vi "Ackermann_FullStochastic_StateSpace.vi"() -> ()   [LabVIEW 2017]
uses:
  <vilib>/Simulation/Scripting/Companion Diagram/SimConfigNode/SimParams.ctl
  <vilib>/Simulation/Scripting/Companion Diagram/SimConfigNode/_simSolvers.ctl
  <vilib>/Simulation/Implementation/Shared/SIMSCR Execution Mode.ctl
  <vilib>/Simulation/Param Hierarchy/Typedefs/SIMPH Param Control Actions.ctl
  <vilib>/Simulation/Implementation/Shared/NILVSim_ParamChanged.vi
  <vilib>/Simulation/Implementation/Shared/NILVSIM_BeginStep.vi
  <vilib>/Simulation/SignalDisplay/Implementation/NILVSim Time Waveform.llb/SIM Time Waveform (vector).vi
  <vilib>/Simulation/Implementation/Shared/NILVSim_Manager.vi
  <vilib>/Utility/error.llb/Clear Errors.vi
  <vilib>/Simulation/Implementation/Shared/NILVSim_FinalizeModel.vi
  <vilib>/Simulation/Implementation/Shared/SIM Unbundle Sim Info.vi
  <vilib>/Simulation/Implementation/Shared/NILVSim_Initialize.vi
  <vilib>/Simulation/Utility/Implementation/NILVSim Get Time and IsAcceptedStep.vi
  <vilib>/Simulation/DiscreteLinear/Implementation/NILVSim Discrete Stochastic State Space.llb/SIM Discrete Stochastic State Space External Indirect Distributor Sim.vi
  <vilib>/Simulation/DiscreteLinear/Implementation/NILVSim Discrete Stochastic State Space.llb/SIM Discrete Stochastic State Space External Indirect Collector Sim.vi
  <vilib>/Simulation/Implementation/Shared/SIMSH Read Queue.vi
  <vilib>/Simulation/Implementation/Shared/NILVSim_GetModelError.vi
  <vilib>/Simulation/Implementation/Shared/SIM Bundle Sim Info.vi
  <vilib>/Simulation/Scripting/Companion Diagram/SimConfigNode/SimDog.xnode
  <vilib>/Simulation/Implementation/XNodeFramework/SimXNode/SimX.xnode
  <vilib>/Simulation/DiscreteLinear/Implementation/NILVSim Discrete Stochastic State Space.llb/NILVSim Discrete Stochastic State Space External Indirect Sim.vi
  <vilib>/Simulation/Implementation/Shared/NI_SIM_Implementation.lvlib
panel:
  out "State Trajectory Graph- Y":cluster{"time":dbl[], dbl[]}[](graph)
  out "State Trajectory Graph- X":cluster{"time":dbl[], dbl[]}[](graph)
  out "State Trajectory Graph- Z":cluster{"time":dbl[], dbl[]}[](graph)
  out "State Trajectory Graph- Phi":cluster{"time":dbl[], dbl[]}[](graph)
  out "State Trajectory Graph- Psi":cluster{"time":dbl[], dbl[]}[](graph)
  out "State Trajectory Graph- Theta":cluster{"time":dbl[], dbl[]}[](graph)
  out "Gain Y":dbl[](array[numeric]) format="%.3f"
  out "Gain X":dbl[](array[numeric]) format="%.3f"
  out "Gain":dbl[](array[numeric]) format="%.3f"
  in  "Phi_rate":dbl
  in  "Theta_rate":dbl
  out "Psi-SSS":picture
  out "Closed-Loop Step Response- Psi":cluster{"time":dbl[], dbl[]}[](graph)
  in  "Imaginary 6":dbl(knob)=-10.013861291935129 scale=0.0..-20.0 scale format="%#_4g"
  in  "Real 6":dbl(knob)=-3.4076115316471642 scale=0.0..-22.0 scale format="%#_4g"
  in  "Psi-Setpoints":dbl[](array[numeric])
  out "State x(k) Psi":dbl[](array[numeric])
  out "Psi":dbl[](array[numeric])
  out "Ux-Phi 4":dbl[](array[numeric]) format="%#.2g"
  out "Waveform Psi":waveform(dbl)[](graph)
  out "theta-SSS":picture
  out "Closed-Loop Step Response- Theta":cluster{"time":dbl[], dbl[]}[](graph)
  in  "Imaginary 5":dbl(knob)=-10.013861291935129 scale=0.0..-20.0 scale format="%#_4g"
  in  "Real 5":dbl(knob)=-3.4076115316471642 scale=0.0..-22.0 scale format="%#_4g"
  out "Theta-Setpoints":dbl[](array[numeric])
  out "State x(k) Theta":dbl[](array[numeric])
  out "Theta":dbl[](array[numeric])
  out "Ux-Phi 3":dbl[](array[numeric]) format="%#.2g"
  out "Waveform Theta":waveform(dbl)[](graph)
  out "Phi-SSS":picture
  out "Closed-Loop Step Response- Phi":cluster{"time":dbl[], dbl[]}[](graph)
  in  "Imaginary 4":dbl(knob)=-10.013861291935129 scale=0.0..-20.0 scale format="%#_4g"
  in  "Real 4":dbl(knob)=-3.4076115316471642 scale=0.0..-22.0 scale format="%#_4g"
  out "Phi-Setpoints":dbl[](array[numeric])
  out "State x(k) Phi":dbl[](array[numeric])
  out "Phi":dbl[](array[numeric])
  out "Ux-Phi 2":dbl[](array[numeric]) format="%#.2g"
  out "Waveform Phi":waveform(dbl)[](graph)
  out "Y-SSS":picture
  out "Closed-Loop Step Response- Y":cluster{"time":dbl[], dbl[]}[](graph)
  in  "Imaginary 3":dbl(knob)=-10.013861291935129 scale=0.0..-20.0 scale format="%#_4g"
  in  "Real 3":dbl(knob)=-3.4076115316471642 scale=0.0..-22.0 scale format="%#_4g"
  in  "Y-Setpoints":dbl[](array[numeric])
  out "State x(k) Y":dbl[](array[numeric])
  out "Y":dbl[](array[numeric])
  out "Uy-Theta":dbl[](array[numeric]) format="%#.2g"
  out "Waveform Y":waveform(dbl)[](graph)
  out "X-SSS":picture
  out "Closed-Loop Step Response- X":cluster{"time":dbl[], dbl[]}[](graph)
  in  "Imaginary 2":dbl(knob)=-10.013861291935129 scale=0.0..-20.0 scale format="%#_4g"
  in  "Real 2":dbl(knob)=-3.4076115316471642 scale=0.0..-22.0 scale format="%#_4g"
  in  "X-Setpoints":dbl[](array[numeric])
  out "State x(k) X":dbl[](array[numeric])
  out "X":dbl[](array[numeric])
  out "Ux-Phi":dbl[](array[numeric]) format="%#.2g"
  out "Waveform X":waveform(dbl)[](graph)
  out "Equation":picture
  in  "reset?":bool
  out "Closed-Loop Step Response":cluster{"time":dbl[], dbl[]}[](graph)
  in  "Imaginary":dbl(knob)=-10.013861291935129 scale=0.0..-20.0 scale format="%#_4g"
  in  "Real":dbl(knob)=-3.4076115316471642 scale=0.0..-22.0 scale format="%#_4g"
  in  "Alt-Setpoints":dbl[](array[numeric])
  out "State x(k) Alt":dbl[](array[numeric])
  out "Altitude":dbl[](array[numeric])
  out "ut":dbl[](array[numeric]) format="%#.2g"
  out "Waveform Altitude":waveform(dbl)[](graph)
  # "I"
  # "R"
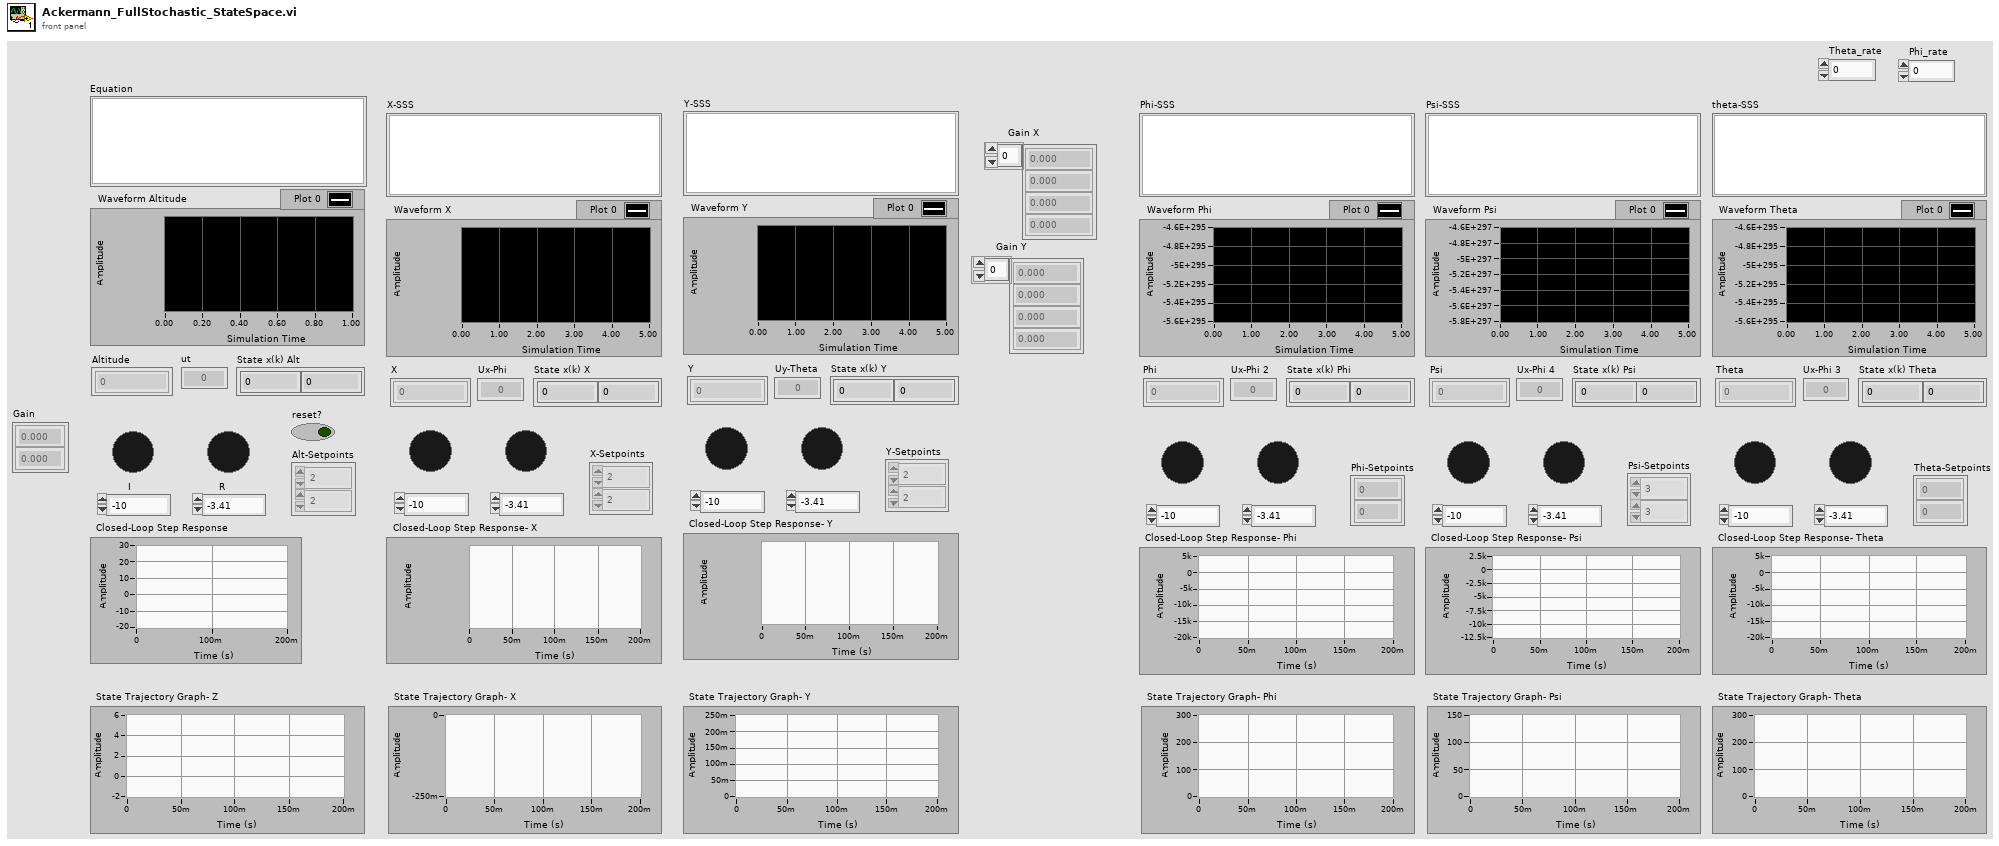
[diagram p1: front panel]
types:
  T1 = typedef "NI_LinSys_Model Typedefs.lvlib/CD State Space Model (MIMO).ctl" = cluster{"properties":T2, "A":dbl[][], "B":dbl[][], "C":dbl[][], "D":dbl[][], "StateNames":string[], "Transport Delay":dbl[][]}
  T2 = typedef "NI_LinSys_Model Typedefs.lvlib/CD General Elements.ctl" = cluster{"Model name":string, "Input names":string[], "Output names":string[], "Input Delays":dbl[], "Output Delays":dbl[], "Sampling Time":dbl, "Notes":string}
  T3 = typedef "NI_CD_Stochastic Systems.lvlib/cd_Stochastic State-Space Model.ctl" = cluster{"Sampling Time (s)":dbl, "G":dbl[][], "B":dbl[][], "A":dbl[][], "C":dbl[][], "D":dbl[][], "H":dbl[][]}
  T4 = typedef "SIMSCR Execution Mode.ctl" = enum16{"Simulate to Completion", "Single Time-Step Simulation (Fixed Step Only)"}
  T5 = typedef "SIMPH Param Control Actions.ctl" = enum16{"get params", "set params"}
  T6 = typedef "SimParams.ctl" = cluster{"Initial Time (s)":dbl, "Final Time (s)":dbl, "Step Size (s)":dbl, "ODE Solver":T7, "Minimum Step Size (s)":dbl, "Maximum Step Size (s)":dbl, "Relative Tolerance":dbl, "Absolute Tolerance":dbl, "Software Timing":bool, "Initial Step Size (s)":dbl, "Automatic Fixed Step Size?":bool, "Automatic Discrete Step Size?":bool, "Discrete Step Size (s)":dbl, "Calculate using Time Step":bool, "Solver Wired?":bool, "Prev.Frm.Expected End":u64, "Prev.Frm.Actual End":u64, "Prev.Frm.Finished Late?":bool, "Prev.Iter.Expected End":u64, "Prev.Iter.Actual End":u64, "Prev.Iter.Finished Late?":bool, "Expected Iteration Start":u64, "Actual Iteration Start":u64, "Expected Frame Start":u64, "Actual Frame Start":u64, "Source Name":string, "Name":string, "Period":i64, "Deadline":i64, "Offset":i64, "Start":i64, "Priority":i32, "Timeout":i32, "Processor":i32, "Mode":enum32{"No Change", "Process missed periods, maintain original phase", "Discard missed periods, maintain original phase", "Process missed periods, ignore original phase", "Discard missed periods, ignore original phase"}, "Wakeup reason":enum32{"Normal", "Aborted", "Asynchronous wakeup", "Timing source error", "Timed loop error", "Timeout"}, "Error":errorcluster, "Source Type":string, "Secondary Source Type":string, "Global End Time":u64, "Global Start Time":u64, "Full Solver Reset":bool, "Execution Mode":T4, "Nan/Inf Check":bool, "Custom Solver Library":string, "Solver Is Variable":bool, "custom solver name":string, "Signal Collection Decimation":u32}
  T7 = typedef "_simSolvers.ctl" = enum16{"Runge-Kutta 1 (Euler)", "Runge-Kutta 2", "Runge-Kutta 3", "Runge-Kutta 4", "Runge-Kutta 23 (variable)", "Runge-Kutta 45 (variable)", "BDF (variable)", "Adams-Moulton (variable)", "Rosenbrock (variable)", "Discrete States Only", "SDIRK 4 (variable)", "Radau 5 (variable)", "Radau 9 (variable)", "Radau 13 (variable)", "Radau [Variable Order] (variable)", "Gear's Method (variable)", "Linearizer", "State Query", "Trim Eval", "Custom Solver"}
  T8 = typedef "NI_LinSys_Data Typedefs.lvlib/CD Parametric Time Response Data.ctl" = cluster{"Rise Time (s)":dbl[][], "Peak Time (s)":dbl[][], "Settling Time (s)":dbl[][], "Overshoot (%)":dbl[][], "Steady-State Gain":dbl[][], "Peak Value":dbl[][]}
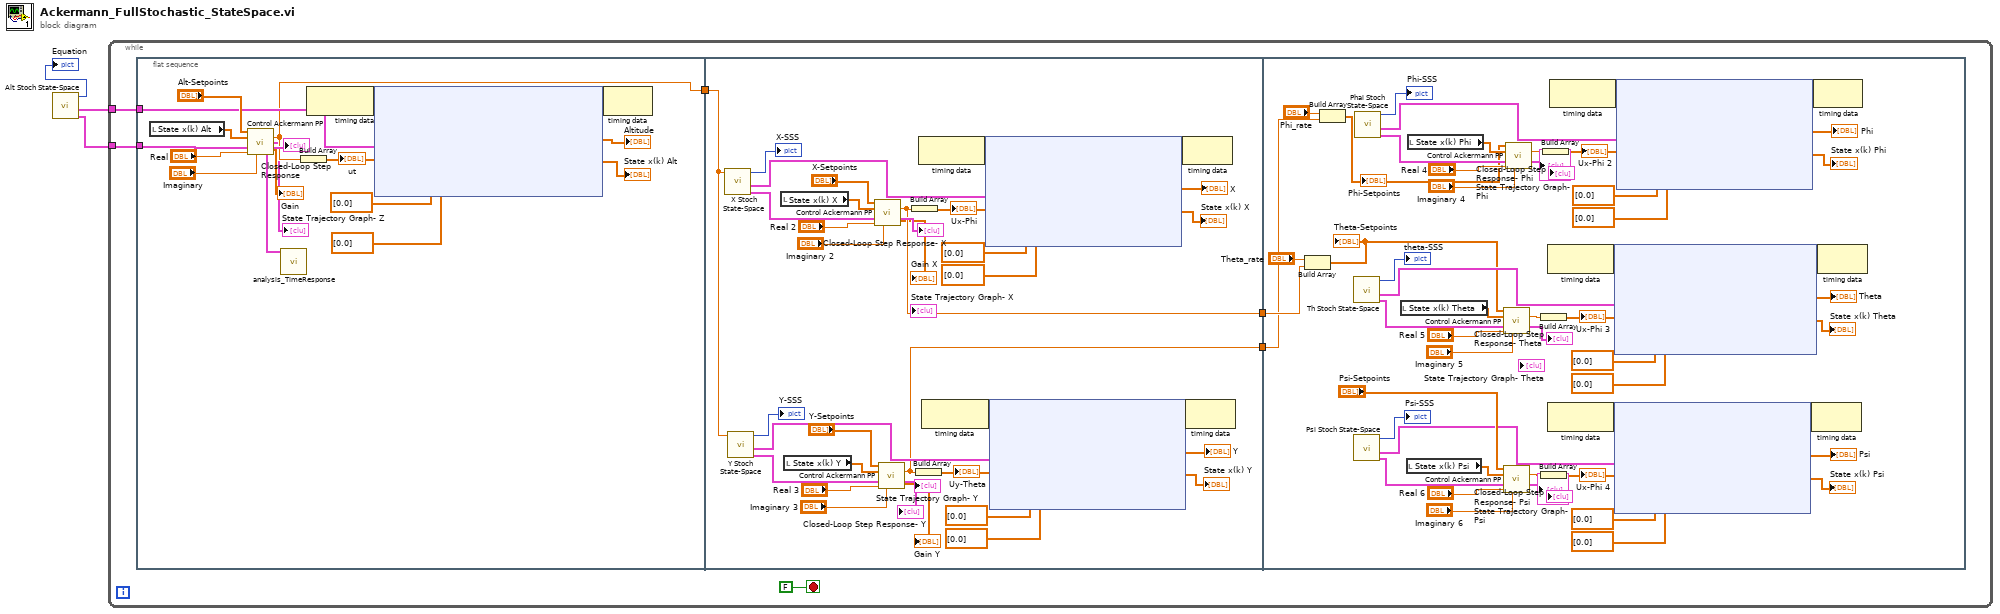
[diagram p0: block diagram]
diagram:
  n1 = call "Alt Stoch State-Space.vi"() -> ("Deterministic Alt State-Space Model"=w3:T1, "Altitude Stochastic State-Space Model"=w2:T3, "Equation"=→"Equation":picture)  [unwired: 5 in, 4 out]
  n2 = while {
    tunnel: w3 -> [w8]
    tunnel: w2 -> [w7]
    stop <- FALSE stop-if-true
    n3 = flat-sequence {
      tunnel: w8 -> [w19]
      tunnel: w7 -> [w16]
      tunnel: [w13] -> w6
      tunnel: w6 -> [w312]
      tunnel: [w311] -> w5
      tunnel: [w310] -> w4
      tunnel: w5 -> [w950]
      tunnel: w4 -> [w949]
      frame #0 {
        n4 = local read "State x(k) Alt"() -> (w21:dbl[])
        n5 = call "Control Ackermann PP.vi"("Setpoints"="Alt-Setpoints", "state x(k)"=w21, "State-Space Model"=w19, "Real"="Real", "Imaginary"="Imaginary") -> ("Controller Action"=w13:dbl, "State Trajectory Graph"=→"State Trajectory Graph- Z":cluster{"time":dbl[], dbl[]}[], "Closed-Loop Step Response"=→"Closed-Loop Step Response":cluster{"time":dbl[], dbl[]}[], "Gain"=→"Gain":dbl[], "Time Response Parametric Data"=w11:T8)  [unwired: 2 in, 4 out]
        n6 = call "analysis_TimeResponse.vi"("Time Response Parametric Data"=w11) -> ()  [unwired: 5 in, 6 out]
        n7 = Build Array(w13) -> (w15:dbl[])
        "ut" <- w15
        n8 = node-c288() -> (w27:variant)  [unwired: 1 in]
        n9 = node-c254 ("Control & Simulation Loop")(w27, dbl[] [0.0] ("Process Noise w(k)"), dbl[] [0.0] ("Measurement Noise v(k)"), w16, w15) -> (w26:variant, →"Altitude":dbl[], →"State x(k) Alt":dbl[])
        n10 = node-c288(w26) -> ()  [unwired: 1 out]
      }
      frame #1 {
        n11 = call "X Stoch State-Space.vi"("ut"=w312) -> ("X Deterministic State-Space Model"=w329:T1, "X Stochastic State-Space Model"=w330:T3, "Equation"=→"X-SSS":picture)  [unwired: 4 in, 4 out]
        n12 = call "Y Stoch State-Space.vi"("ut"=w312) -> ("Y Deterministic State-Space Model"=w314:T1, "Y Stochastic State-Space Model"=w315:T3, "Equation"=→"Y-SSS":picture)  [unwired: 4 in, 4 out]
        n13 = local read "State x(k) X"() -> (w336:dbl[])
        n14 = local read "State x(k) Y"() -> (w321:dbl[])
        n15 = call "Control Ackermann PP.vi"("Setpoints"="X-Setpoints", "state x(k)"=w336, "State-Space Model"=w329, "Real"="Real 2", "Imaginary"="Imaginary 2") -> ("Controller Action"=w311:dbl, "Closed-Loop Step Response"=→"Closed-Loop Step Response- X":cluster{"time":dbl[], dbl[]}[], "Gain"=→"Gain X":dbl[])  [unwired: 2 in, 6 out]
        n16 = call "Control Ackermann PP.vi"("Setpoints"="Y-Setpoints", "state x(k)"=w321, "State-Space Model"=w314, "Real"="Real 3", "Imaginary"="Imaginary 3") -> ("Controller Action"=w310:dbl, "Closed-Loop Step Response"=→"Closed-Loop Step Response- Y":cluster{"time":dbl[], dbl[]}[], "Gain"=→"Gain Y":dbl[])  [unwired: 2 in, 6 out]
        n17 = Build Array(w311) -> (w332:dbl[])
        "Ux-Phi" <- w332
        n18 = Build Array(w310) -> (w317:dbl[])
        "Uy-Theta" <- w317
        n19 = node-c288() -> (w342:variant)  [unwired: 1 in]
        n20 = node-c288() -> (w327:variant)  [unwired: 1 in]
        n21 = node-c254 ("Control & Simulation Loop 2")(w342, dbl[] [0.0] ("Process Noise w(k)"), dbl[] [0.0] ("Measurement Noise v(k)"), w330, w332) -> (w341:variant, →"X":dbl[], →"State x(k) X":dbl[])
        n22 = node-c254 ("Control & Simulation Loop 3")(w327, dbl[] [0.0] ("Process Noise w(k)"), dbl[] [0.0] ("Measurement Noise v(k)"), w315, w317) -> (w326:variant, →"Y":dbl[], →"State x(k) Y":dbl[])
        n23 = node-c288(w341) -> ()  [unwired: 1 out]
        n24 = node-c288(w326) -> ()  [unwired: 1 out]
      }
      frame #2 {
        n25 = Build Array("Theta_rate", w950) -> (w901:dbl[])
        "Theta-Setpoints" <- w901
        n26 = Build Array("Phi_rate", w949) -> (w899:dbl[])
        "Phi-Setpoints" <- w899
        n27 = call "Th Stoch State-Space.vi"() -> ("Theta Deterministic State-Space Model"=w904:T1, "Theta Stochastic State-Space Model"=w919:T3, "Equation"=→"theta-SSS":picture)  [unwired: 5 in, 4 out]
        n28 = call "Psi Stoch State-Space.vi"() -> ("Psi Deterministic State-Space Model"=w903:T1, "Psi Stochastic State-Space Model"=w906:T3, "Equation"=→"Psi-SSS":picture)  [unwired: 5 in, 4 out]
        n29 = call "Phai Stoch State-Space.vi"() -> ("Phi Deterministic State-Space Model"=w931:T1, "Phai Stochastic State-Space Model"=w932:T3, "Equation"=→"Phi-SSS":picture)  [unwired: 5 in, 4 out]
        n30 = local read "State x(k) Theta"() -> (w925:dbl[])
        n31 = local read "State x(k) Psi"() -> (w913:dbl[])
        n32 = local read "State x(k) Phi"() -> (w938:dbl[])
        n33 = call "Control Ackermann PP.vi"("Setpoints"=w901, "state x(k)"=w925, "State-Space Model"=w904, "Real"="Real 5", "Imaginary"="Imaginary 5") -> ("Controller Action"=w922:dbl, "Closed-Loop Step Response"=→"Closed-Loop Step Response- Theta":cluster{"time":dbl[], dbl[]}[])  [unwired: 2 in, 7 out]
        n34 = call "Control Ackermann PP.vi"("Setpoints"="Psi-Setpoints", "state x(k)"=w913, "State-Space Model"=w903, "Real"="Real 6", "Imaginary"="Imaginary 6") -> ("Controller Action"=w909:dbl, "Closed-Loop Step Response"=→"Closed-Loop Step Response- Psi":cluster{"time":dbl[], dbl[]}[])  [unwired: 2 in, 7 out]
        n35 = call "Control Ackermann PP.vi"("Setpoints"=w899, "state x(k)"=w938, "State-Space Model"=w931, "Real"="Real 4", "Imaginary"="Imaginary 4") -> ("Controller Action"=w935:dbl, "Closed-Loop Step Response"=→"Closed-Loop Step Response- Phi":cluster{"time":dbl[], dbl[]}[])  [unwired: 2 in, 7 out]
        n36 = Build Array(w922) -> (w921:dbl[])
        "Ux-Phi 3" <- w921
        n37 = Build Array(w909) -> (w908:dbl[])
        "Ux-Phi 4" <- w908
        n38 = Build Array(w935) -> (w934:dbl[])
        "Ux-Phi 2" <- w934
        n39 = node-c288() -> (w946:variant)  [unwired: 1 in]
        n40 = node-c288() -> (w944:variant)  [unwired: 1 in]
        n41 = node-c288() -> (w948:variant)  [unwired: 1 in]
        n42 = node-c254 ("Control & Simulation Loop 5")(w946, dbl[] [0.0] ("Process Noise w(k)"), dbl[] [0.0] ("Measurement Noise v(k)"), w919, w921) -> (w945:variant, →"Theta":dbl[], →"State x(k) Theta":dbl[])
        n43 = node-c254 ("Control & Simulation Loop 6")(w944, dbl[] [0.0] ("Process Noise w(k)"), dbl[] [0.0] ("Measurement Noise v(k)"), w906, w908) -> (w943:variant, →"Psi":dbl[], →"State x(k) Psi":dbl[])
        n44 = node-c254 ("Control & Simulation Loop 4")(w948, dbl[] [0.0] ("Process Noise w(k)"), dbl[] [0.0] ("Measurement Noise v(k)"), w932, w934) -> (w947:variant, →"Phi":dbl[], →"State x(k) Phi":dbl[])
        n45 = node-c288(w943) -> ()  [unwired: 1 out]
        n46 = node-c288(w947) -> ()  [unwired: 1 out]
        n47 = node-c288(w945) -> ()  [unwired: 1 out]
      }
    }
  }
